vi "Get Programmer Settings.vi"(8 "Programmer Type":string, 9 "Chip":string, 11 "Test Template in":refnum<class "Program Driver.lvclass">) -> (3 "Programmer Settings":string[](array[string]))   [LabVIEW 2015, in "Program Driver.lvclass"]
uses:
  Program Driver.lvclass
  Test Class/Test Class.lvclass
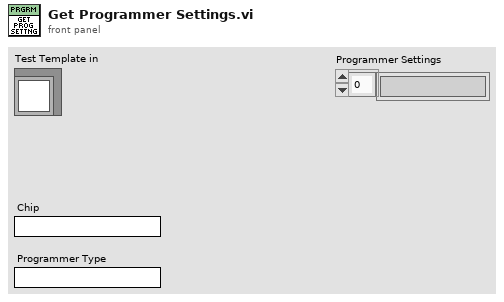
[diagram p1: front panel]
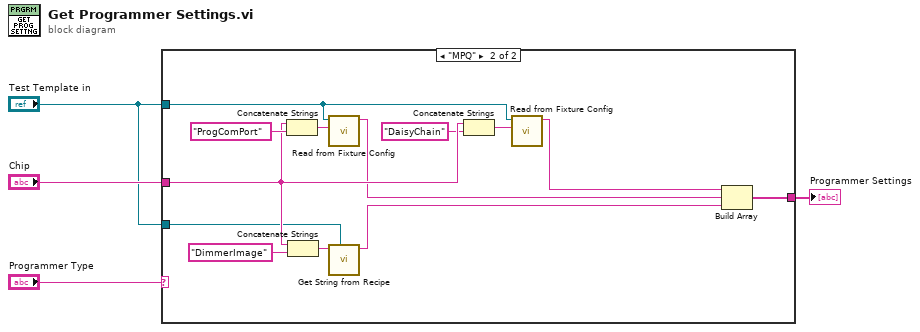
[diagram p0: block diagram]
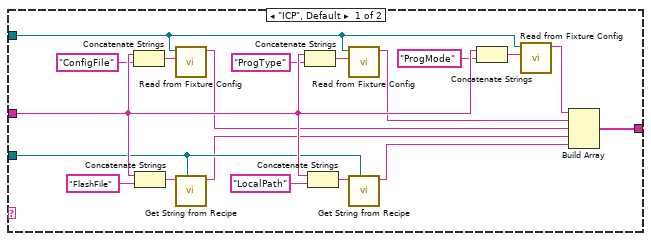
[diagram p2: hidden frame]
diagram:
  n1 = case shown="\"MPQ\"" "Programmer Type" {
    tunnel: "Chip" -> [w23 w34]
    tunnel: "Test Template in" -> [w10 w32]
    tunnel: "Test Template in" -> [w8 w26]
    tunnel: [w17 w33] -> w3
    frame "ICP", Default {
      n2 = Concatenate Strings(w23, "ConfigFile" ("String")) -> (w15:string)
      n3 = Concatenate Strings(w23, "FlashFile" ("String")) -> (w5:string)
      n4 = call-dynamic "Read from Fixture Config.vi"("Key"=w15, "Test Class in"=w10) -> ("Instrument Info"=w16:string)  [unwired: 8 in, 1 out]
      n5 = call "Get String from Recipe.vi"("Test Class in"=w8, "Name"=w5) -> ("Value"=w7:string)  [unwired: 7 in, 2 out]
      n6 = Concatenate Strings(w23, "ProgType" ("String")) -> (w14:string)
      n7 = Concatenate Strings(w23, "LocalPath" ("String")) -> (w9:string)
      n8 = call-dynamic "Read from Fixture Config.vi"("Key"=w14, "Test Class in"=w10) -> ("Instrument Info"=w13:string)  [unwired: 8 in, 1 out]
      n9 = call "Get String from Recipe.vi"("Test Class in"=w8, "Name"=w9) -> ("Value"=w6:string)  [unwired: 7 in, 2 out]
      n10 = Concatenate Strings(w23, "ProgMode" ("String")) -> (w12:string)
      n11 = call-dynamic "Read from Fixture Config.vi"("Key"=w12, "Test Class in"=w10) -> ("Instrument Info"=w11:string)  [unwired: 8 in, 1 out]
      n12 = Build Array(w11, w13, w16, w7, w6) -> (w17:string[])
    }
    frame "MPQ" {
      n13 = Concatenate Strings(w34, "ProgComPort" ("String")) -> (w27:string)
      n14 = Concatenate Strings(w34, "DimmerImage" ("String")) -> (w25:string)
      n15 = call-dynamic "Read from Fixture Config.vi"("Key"=w27, "Test Class in"=w32) -> ("Instrument Info"=w28:string)  [unwired: 8 in, 1 out]
      n16 = call "Get String from Recipe.vi"("Test Class in"=w26, "Name"=w25) -> ("Value"=w24:string)  [unwired: 7 in, 2 out]
      n17 = Concatenate Strings(w34, "DaisyChain" ("String")) -> (w30:string)
      n18 = call-dynamic "Read from Fixture Config.vi"("Key"=w30, "Test Class in"=w32) -> ("Instrument Info"=w29:string)  [unwired: 8 in, 1 out]
      n19 = Build Array(w29, w28, w24) -> (w33:string[])
    }
  }
  "Programmer Settings" <- w3
